vi "Dashboard Main.vi"() -> ()   [LabVIEW 2014]
uses:
  <vilib>/event_ctls.llb/eventvkey.ctl
  <vilib>/Rock Robotics/WPI/Dashboard/WPI_DashboardLogging Global.vi
  <vilib>/Rock Robotics/Network Tables/SD Write Numeric Array.vi
  <vilib>/Rock Robotics/Network Tables/SD Write String.vi
  <vilib>/Rock Robotics/Network Tables/SD Read Number.vi
  <vilib>/Utility/config.llb/Write Key (String).vi
  <vilib>/Utility/config.llb/Write Key (I32).vi
  <vilib>/Utility/config.llb/NI_LVConfig.lvlib
panel:
  in  "TCP":refnum<k5>
  in  "Rec Mode":enum32{"Stop", "Record", "Playback"}(radio)
  in  "Vision":u16(ring) items=["Camera Off", "USB Camera SW", "USB Camera HW", "IP Camera"]
  out "Camera IP":string
  out "Image Message":string="Timeout in Camera Communications"
  in  "Dashboard Tab":T1(tab)
  in  "Camera Settings":T2={"Frame Rate"=30, "Compression"=30, "Size"=1} {"Frame Rate" scale=1.0..30.0; "Size" items=["640x480", "320x240", "160x120"]}
  out "MotorChart R":cluster{"Numeric":dbl, "Numeric":dbl}(graph)
  out "MotorChart L":T3(graph)
  out "MotorSliders R":cluster{"MotorSlide1":dbl, "MotorSlide2":dbl} {"MotorSlide2" scale=-1.0..1.0 scale format="%#_2e"; "MotorSlide1" scale=-1.0..1.0 scale format="%#_2e"}
  out "MotorSliders L":T4 {"MotorSlide4 2" scale=0.0..14.0 scale format="%#_2e"; "MotorSlide2" scale=-1.0..1.0 scale format="%#_2e"; "MotorSlide1" scale=-1.0..1.0 scale format="%#_2e"}
  out "Gyro":dbl(knob) scale=0.0..360.0
  out "JS1 Z":dbl(slide) scale=-1.0..1.0 scale format="%#_2e"
  out "JS1 Graph":cluster{"X":dbl, "Y":dbl}[](graph)
  out "JS1 Buttons":T5
  out "JS2 Z":dbl(slide) scale=-1.0..1.0 scale format="%#_2e"
  out "JS2 Graph":cluster{"X":dbl, "Y":dbl}[](graph)
  out "JS2 Buttons":T5
  out "Mode":T6(ring)=enum."Auto Disabled"
  in  "DB Camera Config":bool
  out "fps":dbl format="%#.1g"
  out "Mbps":dbl format="%#.1g"
  out "Mbps 2":bool
  in  "DB/String 9":string
  in  "DB/String 8":string
  in  "DB/String 7":string
  in  "DB/String 6":string
  in  "DB/String 5":string
  in  "DB/String 4":string
  in  "DB/String 3":string
  in  "DB/String 2":string
  in  "DB/String 1":string
  in  "DB/String 0":string
  in  "DB/Slider 0":dbl(slide) scale=0.0..5.0
  in  "DB/Slider 1":dbl(slide) scale=0.0..5.0
  in  "DB/Slider 2":dbl(slide) scale=0.0..5.0
  in  "DB/Slider 3":dbl(slide) scale=0.0..5.0
  out "DB/LED 3":bool
  out "DB/LED 2":bool
  out "DB/LED 1":bool
  out "DB/LED 0":bool
  in  "DB/Button 3":bool
  in  "DB/Button 2":bool
  in  "DB/Button 1":bool
  in  "DB/Button 0":bool caption="New Name"
  in  "Turning Speed":dbl
  in  "Initial turn (Degrees)":dbl
  in  "Move Speed":dbl
  in  "Arm Speed":dbl
  in  "Shifting Speed":dbl
  in  "Desired Arm height (Lift)":dbl
  in  "Desired Arm height (Lowered)":dbl
  in  "Shifting time (Initial)":dbl
  in  "Auto Mode":string(combo)
  in  "Test Slider":dbl(slide) scale=0.0..100.0 scale format="%#_3g"
  in  "On/Off":bool caption="Solenoid"
  in  "Test Name":u16(ring) items=["Select the test to run...", "Example Test", "-------------------------------", "List of tests is built in robot code.", "Replace with your own automated tests."]
  in  "Test Tree":string(tree)
  in  "Motor":cluster{"Value":dbl, "Enable":bool} {"Value" scale=-1.0..1.0 scale format="%#_3g"}
  out "Progress":T7 {"Test Progress" scale=0.0..100.0}
  in  "Rev/Fwd":cluster{"Forward":bool, "Reverse":bool}
  in  "Test Ring":u16(ring) items=["Monochrome", "Color"]
  in  "Listbox":i32(listbox)
  out "Tree":string(tree)
  out "Camera Image":T8(plugin-control)
  out "Boolean":bool
  # "Left"
  # "Front"
  # "Right"
  # "Battery"
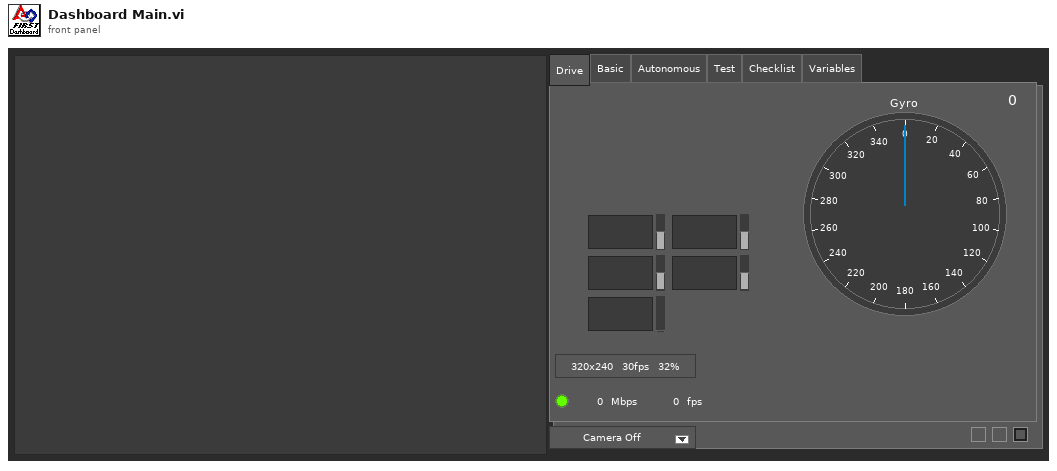
[diagram p1: front panel]
types:
  T1 = enum32{"Drive", "Basic", "Autonomous", "Test", "Checklist", "Variables"}
  T2 = cluster{"Frame Rate":i32, "Compression":i32, "Size":u16}
  T3 = cluster{"Numeric":dbl, "Numeric":dbl, "Battery V":dbl}
  T4 = cluster{"MotorSlide1":dbl, "MotorSlide2":dbl, "MotorSlide4 2":dbl}
  T5 = cluster{bool, bool, bool, bool, bool, bool, bool, bool, bool, bool, bool, bool}
  T6 = enum8{"Tele-Op Disabled", "Tele-Op Enabled", "Auto Disabled", "Auto Enabled", "Test Disabled", "Test Enabled", "Disconnected", "No Code", "E-Stop"}
  T7 = cluster{"Test Progress":u8, "Test Progress Text":string}
  T8 = typedef "IMAQ Image.ctl" = refnum<image>
  T9 = enum32{"Drive", "Basic", "Custom", "Test", "Checklist", "Variables"}
  T10 = typedef "Image Type" = u32
  T11 = cluster{"Camera Image":refnum<vi>, "Dashboard Tab":refnum<vi>, "Boolean":refnum<vi>, "Vision":refnum<vi>, "Rec Mode":refnum<vi>, "Test Slider":refnum<vi>, "On/Off ":refnum<vi>, "Test Ring":refnum<vi>, "Rev/Fwd":refnum<vi>, "Test Name":refnum<vi>, "Motor":refnum<vi>, "Progress":refnum<vi>, "CheckList":refnum<vi>, "Tree":refnum<vi>, "Test Tree":refnum<vi>}
  T12 = cluster{"Error Strings":string, "Disable Counts":cluster{u16, u16}, "Rail Faults":cluster{u16, u16, u16}, "Robot IP":string, "DB Mode":u8, "Event Info":cluster{"Name":string, "Type":u8, "Number":u16, "Replay":u8}, "Camera Addr":string}
  T13 = cluster{"Storage":cluster{"Disk Free":u64, "RAM Block":u32, "RAM free":u32}, "CPU Utilization":cluster{"CPU % ISR":sgl, "CPU % Time Crit":sgl, "CPU % Timed Str":sgl, "CPU % High":sgl, "CPU % Above":sgl, "CPU % Normal":sgl, "CPU % Low":sgl}, "CAN":cluster{"% Bus Utilization":sgl, "Bus Off Cnt":u32, "TX_FIFO Full Cnt":u32, "Receive Error Cnt":u8, "Transmit Error Cnt":u8}, "HID":cluster{"HID Outputs":u32, "Rumble Low":u16, "Rumble High":u16}[]}
  T14 = cluster{"Status bits":cluster{"Test Mode":bool, "Autonomous":bool, "Enabled":bool, "Code Start":bool, "Brownout":bool, "Reserved 2":bool, "Reserved 3":bool, "E-Stop":bool}, "Code Trace":cluster{"Disabled":bool, "TeleOp":bool, "Auto":bool, "Test":bool}, "Controller Type":enum16{"unknown", "cRIO", "roboRio"}, "Code?":enum16{"unknown", "noCode", "code"}, "Battery V":dbl}
  T15 = cluster{"Control Bits":cluster{"TestMode":bool, "Autonomous":bool, "Enabled":bool, "FMS Present":bool, bool, bool, bool, "E-Stop":bool}, "Team Station ":u8, "Countdown":sgl, "Joystick Values":cluster{"Axes":dbl[], "Buttons":bool[], "POVs":i16[]}[]}
  T16 = cluster{"Axes":dbl[], "Buttons":bool[], "POVs":i16[]}[]
  T17 = cluster{"Axes":dbl[], "Buttons":bool[], "POVs":i16[]}
  T18 = cluster{"Buttons[0]":bool, "Buttons[1]":bool, "Buttons[2]":bool, "Buttons[3]":bool, "Buttons[4]":bool, "Buttons[5]":bool, "Buttons[6]":bool, "Buttons[7]":bool, "Buttons[8]":bool, "Buttons[9]":bool, "Buttons[10]":bool, "Buttons[11]":bool}
  T19 = typedef "NI_LVConfig.lvlib/Config Data RefNum.ctl" = refnum<k1>
  T20 = cluster{"Operation":enum16{"Update", "Clear"}, "Color Box":u32}[]
  T21 = typedef "eventvkey.ctl" = enum16{"ASCII", "Enter", "Return", "Shift", "Ctrl", "Alt", "Cmd", "Opt", "Caps", "NumLock", "Clear", "Break", "Up", "Down", "Left", "Right", "Insert", "Delete", "Home", "End", "PageUp", "PageDown", "Escape", "Help", "Pause", "ScrollLock", "F1", "F2", "F3", "F4", "F5", "F6", "F7", "F8", "F9", "F10", "F11", "F12", "F13", "F14", "F15", "F16", "F17", "F18", "F19", "F20", "F21", "F22", "F23", "F24", "Play", "VolumeUp", "VolumeDown", "Mute", "Two Byte Char"}
  T22 = cluster{"Image Size":bool, "Image Type":bool, "Pixel Value":bool, "ROI Information":bool, "Zoom Factor":bool}
  T23 = enum8{"Enabled", "Disabled", "Disabled and Grayed Out"}
  T24 = cluster{"Operation":enum16{"Update", "Clear"}, "Color Box":u32}
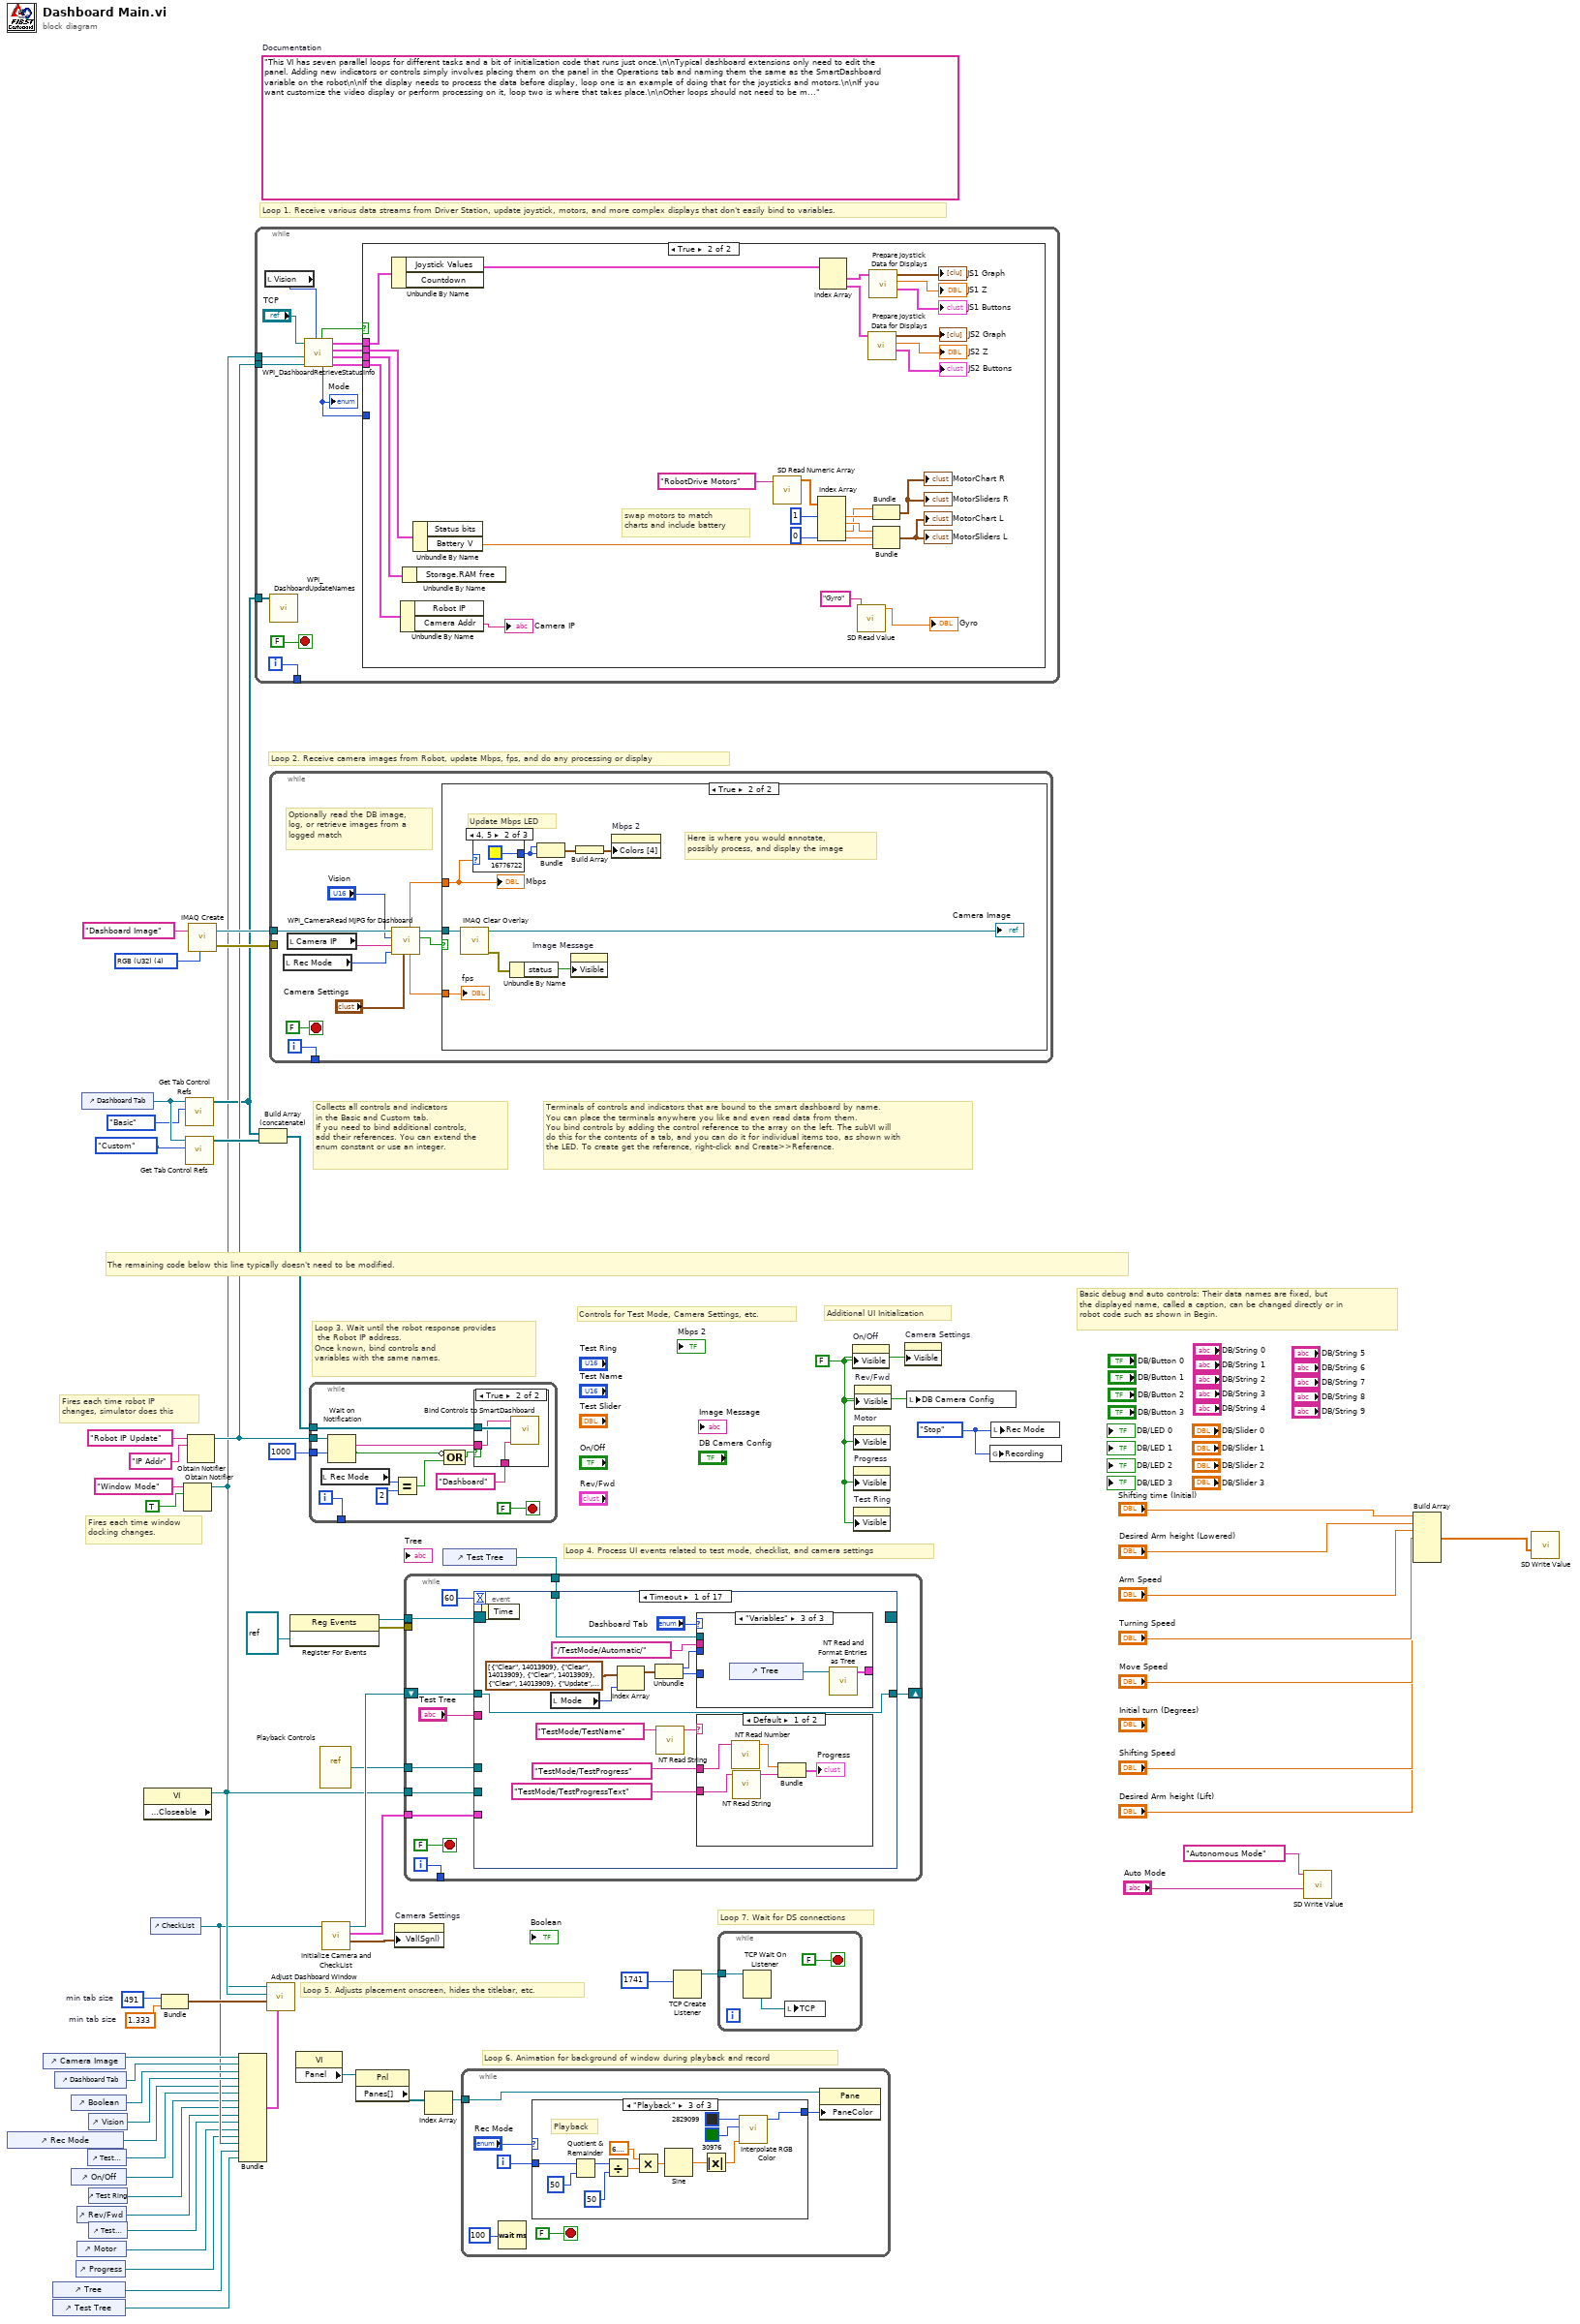
[diagram p0: block diagram]
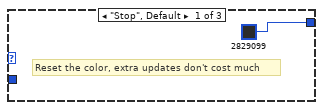
[diagram p3: hidden frame]
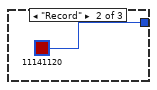
[diagram p4: hidden frame]
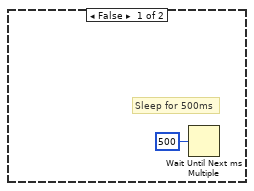
[diagram p6: hidden frame]
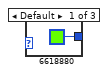
[diagram p7: hidden frame]
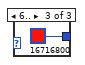
[diagram p8: hidden frame]
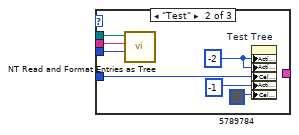
[diagram p10: hidden frame]
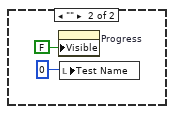
[diagram p11: hidden frame]
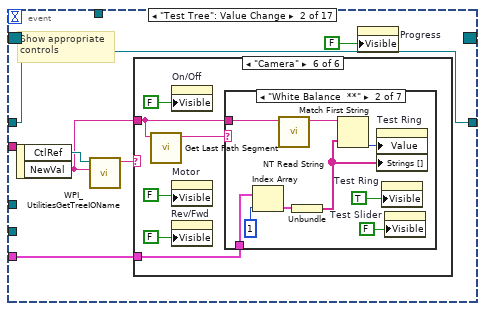
[diagram p12: hidden frame]
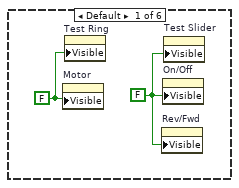
[diagram p13: hidden frame]
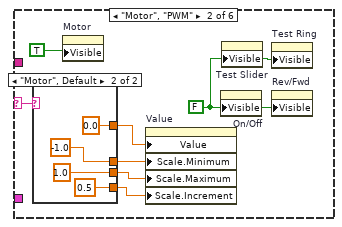
[diagram p14: hidden frame]
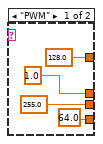
[diagram p15: hidden frame]
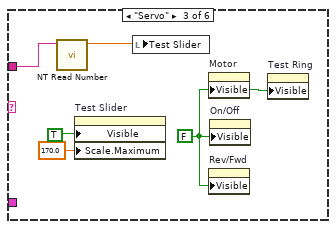
[diagram p16: hidden frame]
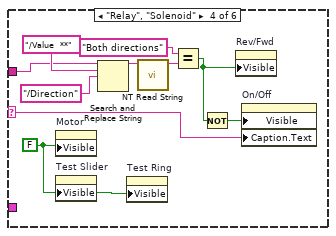
[diagram p17: hidden frame]
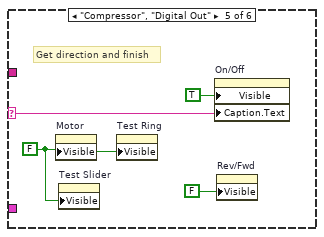
[diagram p18: hidden frame]
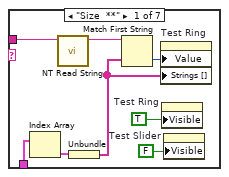
[diagram p19: hidden frame]
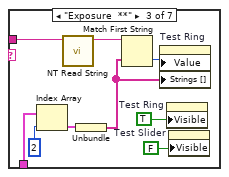
[diagram p20: hidden frame]
diagram:
  w34 = 491  # min tab size
  w33 = 1.333  # min tab size
  w42 = enum32{"Stop", "Record", "Playback"}."Stop" ("Rec Mode")
  w16 = FALSE ("Visible")
  (unwired) "This VI has seven parallel loops for different tasks and a bit of initialization code that runs just once.\n\nTypical dashboard extensions only need to edit the panel. Adding new indicators or controls simply involves placing them on the panel in the Operations tab and naming them the same as the SmartDashboard variable on the robot\n\nIf the display needs to process the data before display, loop one is an example of doing that for the joysticks and motors.\n\nIf you want customize the video display or perform processing on it, loop two is where that takes place.\n\nOther loops should not need to be modified. They are pretty standard, and document the task they perform."  # Documentation
  w62 = T10 4 items=["Grayscale (U8)", "Grayscale (I16)", "Grayscale (SGL)", "Complex (CSG)", "RGB (U32)", "HSL (U32)", "RGB (U64)"] ("Image Type")
  # "Loop 7. Wait for DS connections"
  # "Basic debug and auto controls: Their data names are fixed, but\nthe displayed name, called a caption, can be changed directly or in\nrobot code such as shown in Begin."
  # "Controls for Test Mode, Camera Settings, etc."
  # "Additional UI Initialization"
  # "Loop 6. Animation for background of window during playback and record"
  # "Fires each time robot IP\nchanges, simulator does this"
  # "Fires each time window\ndocking changes."
  # "Collects all controls and indicators\nin the Basic and Custom tab.\nIf you need to bind additional controls,\nadd their references. You can extend the\nenum constant or use an integer."
  # "The remaining code below this line typically doesn't need to be modified."
  # "Loop 4. Process UI events related to test mode, checklist, and camera settings"
  # "Terminals of controls and indicators that are bound to the smart dashboard by name.\nYou can place the terminals anywhere you like and even read data from them.\nYou bind controls by adding the control reference to the array on the left. The subVI will\ndo this for the contents of a tab, and you can do it for individual items too, as shown with\nthe LED. To create get the reference, right-click and Create>>Reference."
  # "Loop 3. Wait until the robot response provides\n the Robot IP address.\nOnce known, bind controls and\nvariables with the same names."
  # "Loop 5. Adjusts placement onscreen, hides the titlebar, etc."
  # "Loop 1. Receive various data streams from Driver Station, update joystick, motors, and more complex displays that don't easily bind to variables."
  # "Loop 2. Receive camera images from Robot, update Mbps, fps, and do any processing or display"
  n1 = control-ref of="Rec Mode"() -> (w22:refnum<vi>)
  n2 = control-ref of="Camera Image"() -> (w37:refnum<vi>)
  n3 = control-ref of="Tree"() -> (w26:refnum<vi>)
  n4 = control-ref of="Test Tree"() -> (w25:refnum<vi>)
  n5 = control-ref of="Dashboard Tab"() -> (w36:refnum<vi>)
  n6 = control-ref of="Boolean"() -> (w31:refnum<vi>)
  n7 = control-ref of="On/Off"() -> (w20:refnum<vi>)
  n8 = control-ref of="Progress"() -> (w17:refnum<vi>)
  n9 = control-ref of="Rev/Fwd"() -> (w18:refnum<vi>)
  n10 = control-ref of="Motor"() -> (w23:refnum<vi>)
  n11 = control-ref of="Dashboard Tab"() -> (w40:refnum<vi>)
  n12 = control-ref of="Test Slider"() -> (w21:refnum<vi>)
  n13 = control-ref of="Vision"() -> (w35:refnum<vi>)
  n14 = control-ref of="Test Ring"() -> (w19:refnum<vi>)
  n15 = control-ref of="Test Name"() -> (w24:refnum<vi>)
  n16 = property class="VI" props=["Front Panel.Closeable"]() -> (reference out=w41:refnum<vi>)  [unwired: 2 in, 2 out]
  n17 = control-ref of="CheckList"() -> (w27:refnum<vi>)
  n18 = Bundle("min tab size"=w34, "min tab size"=w33) -> (w32:cluster{"min tab size":i32, "min tab size":dbl})  [unwired: 1 in]
  n19 = Obtain Notifier(name (unnamed)="Window Mode", notification data type=TRUE) -> (notifier out=w13:refnum<notifier>)  [unwired: 2 in, 2 out]
  n20 = call <vilib>:"Get Tab Control Refs.vi"("Page Index"=T9."Basic" ("Dashboard Tab"), "TabControl in"=w40) -> ("ControlsOnPage"=w14:refnum<vi>[])  [unwired: 9 in]
  n21 = call <vilib>:"Get Tab Control Refs.vi"("Page Index"=T9."Custom" ("Dashboard Tab"), "TabControl in"=w40) -> ("ControlsOnPage"=w39:refnum<vi>[])  [unwired: 9 in]
  n22 = Obtain Notifier(name (unnamed)="Robot IP Update", notification data type="IP Addr" ("name (unnamed)")) -> (notifier out=w15:refnum<notifier>)  [unwired: 2 in, 2 out]
  n23 = call "IMAQ Create"("Image Name"="Dashboard Image", "Image Type"=w62) -> ("New Image"=w60:T8, "error out"=w59:errorcluster)  [unwired: 2 in, 1 out]
  n24 = Bundle("Camera Image"=w37, "Dashboard Tab"=w36, "Boolean"=w31, "Vision"=w35, "Rec Mode"=w22, "Test Slider"=w21, "On/Off"=w20, "Test Ring"=w19, "Rev/Fwd"=w18, "Test Name"=w24, "Motor"=w23, "Progress"=w17, "CheckList"=w27, "Tree"=w26, "Test Tree"=w25) -> (w28:T11)  [unwired: 1 in]
  n25 = while {
    tunnel: [w74] -> _
    tunnel: w15 -> [w68]
    tunnel: w14 -> [w67]
    tunnel: w13 -> [w63]
    i -> [w74]
    stop <- FALSE stop-if-true
    n26 = local read "Vision"() -> (w65:u16)
    n27 = call <vilib>:"WPI_DashboardUpdateNames.vi"("Controls on Tab"=w67) -> ()  [unwired: 11 in]
    n28 = call <vilib>:"WPI_DashboardRetrieveStatusInfo.vi"("Vision"=w65, "Binding Refnum"=w68, "Window Mode Notifier"=w63, "TCP Cnx"="TCP") -> ("Power and Errors"=w69:T12, "Robot Metrics"=w72:T13, "Status Info"=w73:T14, "Control Info"=w70:T15, "Robot Mode"=w66:T6, "Process?"=w71:bool)  [unwired: 2 in]
    "Mode" <- w66
    n29 = case shown="True" w71 {
      tunnel: w73 -> [_ w102]
      tunnel: w72 -> [_ w101]
      tunnel: w70 -> [_ w100]
      tunnel: w69 -> [_ w99]
      tunnel: w66 -> [_ _]
      frame False {
      }
      frame True {
        # "swap motors to match\ncharts and include battery"
        n30 = Unbundle By Name(w100) -> ("Joystick Values"=w87:T16)  [unwired: 1 out]
        n31 = Unbundle By Name(w99) -> ("Camera Addr"=→"Camera IP":string)  [unwired: 1 out]
        n32 = Unbundle By Name(w101) -> ()  [unwired: 1 out]
        n33 = Unbundle By Name(w102) -> ("Battery V"=w88:dbl)  [unwired: 1 out]
        n34 = call <vilib>:"SD Read Numeric Array.vi"("Name"="RobotDrive Motors") -> ("Numeric Array"=w90:dbl[])  [unwired: 8 in, 2 out]
        n35 = Index Array(array=w90, index #1=1, index #4=0) -> (element #1=w94:dbl, element #2=w95:dbl, element #3=w93:dbl, element #4=w98:dbl)  [unwired: 2 in]
        n36 = Index Array(array=w87) -> (element #1=w86:T17, element #2=w81:T17)  [unwired: 2 in]
        n37 = call-poly <vilib>:"SD Read Value.vi"("Name"="Gyro") -> ("Numeric"=→"Gyro":dbl)  [unwired: 8 in, 2 out]
        n38 = call "Prepare Joystick Data for Displays.vi"("Joystick Values"=w81) -> ("Buttons"=→"JS2 Buttons":T18, "Z Axis"=→"JS2 Z":dbl, "Cartesian Data"=→"JS2 Graph":cluster{"X axis":dbl, "X axis":dbl}[])  [unwired: 8 in]
        n39 = call "Prepare Joystick Data for Displays.vi"("Joystick Values"=w86) -> ("Buttons"=→"JS1 Buttons":T18, "Z Axis"=→"JS1 Z":dbl, "Cartesian Data"=→"JS1 Graph":cluster{"X axis":dbl, "X axis":dbl}[])  [unwired: 8 in]
        n40 = Bundle("Numeric"=w93, "Numeric"=w94) -> (→"MotorChart R" →"MotorSliders R":cluster{"Numeric":dbl, "Numeric":dbl})  [unwired: 1 in]
        n41 = Bundle("Numeric"=w95, "Numeric"=w98, "Battery V"=w88) -> (→"MotorChart L" →"MotorSliders L":T3)  [unwired: 1 in]
      }
    }
  }
  n42 = Build Array (concatenate)(w14, w39) -> (w38:refnum<vi>[])
  n43 = call "Adjust Dashboard Window.vi"("Sizing Refnums"=w28, "Size Constraints"=w32, "VI"=w41, "Notifier in"=w13) -> ()  [unwired: 8 in]
  n44 = while {
    tunnel: w60 -> [w111]
    tunnel: w59 -> [_]
    tunnel: [w112] -> _
    i -> [w112]
    stop <- FALSE stop-if-true
    # "Optionally read the DB image,\nlog, or retrieve images from a\nlogged match"
    n45 = local read "Rec Mode"() -> (w105:enum32{"Stop", "Record", "Playback"})
    n46 = local read "Camera IP"() -> (w103:string)
    n47 = call <vilib>:"WPI_CameraRead MJPG for Dashboard.vi"("Camera Settings"="Camera Settings", "Rec Mode"=w105, "Camera IP"=w103, "Camera Mode"="Vision", "Refnum in"=w111) -> ("Active"=w109:bool, "Refnum out"=w110:T8, "FPS"=w108:dbl, "Bandwidth (Mbps)"=w107:dbl)  [unwired: 3 in]
    n48 = case shown="True" w109 {
      tunnel: w110 -> [_ w118]
      tunnel: w107 -> [_ w117]
      tunnel: w108 -> [_ w115]
      frame False {
        # "Sleep for 500ms"
        n49 = Wait Until Next ms Multiple(millisecond multiple=u32 500) -> ()  [unwired: 1 out]
      }
      frame True {
        # "Here is where you would annotate,\npossibly process, and display the image"
        # "Update Mbps LED"
        n50 = call "IMAQ Clear Overlay"("Image"=w118) -> ("error out"=w122:errorcluster, "Image Out"=→"Camera Image":T8)  [unwired: 2 in, 7 out]
        n51 = case shown="4, 5" w117 {
          tunnel: [u32 6618880 ("Color Box") u32 16776722 ("Color Box") u32 16716800 ("Color Box")] -> w119
          frame Default {
          }
          frame 4, 5 {
          }
          frame 6.. {
          }
        }
        n52 = Unbundle By Name(w122) -> ("status"=w123:bool)
        n53 = Bundle("Color Box"=w119, "Color Box"=w119) -> (w121:cluster{"Color Box":u32, "Color Box":u32})  [unwired: 1 out]
        n54 = property on="Image Message" class="Str"("Visible"=w123) -> ()  [unwired: 2 in, 2 out]
        n55 = Build Array(w121) -> (w120:cluster{"Color Box":u32, "Color Box":u32}[])
        n56 = property on="Mbps 2" class="Bool (strict)"("Colors [4]"=w120) -> ()  [unwired: 2 in, 2 out]
        "Mbps" <- w117
        "fps" <- w115
      }
    }
  }
  n57 = register-events(refnum<vi> refnum) -> (reference out=w46:refnum<event-registration>, error out=w45:errorcluster)  [unwired: 2 in]
  n58 = property class="VI"() -> ("Panel"=w49:refnum<vi>)  [unwired: 2 in, 2 out]
  n59 = while {
    tunnel: w38 -> [w138]
    tunnel: w15 -> [w136]
    tunnel: [w134] -> _
    tunnel: u32 1000 ("milliseconds to wait") -> [w133]
    i -> [w134]
    stop <- FALSE stop-if-true
    n60 = local read "Rec Mode"() -> (w129:enum32{"Stop", "Record", "Playback"})
    n61 = Wait on Notification(notifier=w136, timeout in ms (-1)=w133) -> (notification=w135:string, timed out?=w131:bool)  [unwired: 2 in, 2 out]
    n62 = Equal?(x=w129, y=u16 2 ("Rec Mode")) -> (x = y?=w130:bool)
    n63 = Compound Arithmetic op=OR(invert w131, w130) -> (w132:bool)
    n64 = case shown="True" w132 {
      tunnel: w138 -> [_ w141]
      tunnel: w135 -> [_ w140]
      tunnel: "Dashboard" -> [_ w139]
      frame False {
      }
      frame True {
        n65 = call <vilib>:"Bind Controls to SmartDashboard.vi"("Client Name"=w139, "Bound Control Refs"=w141, "Server IP Address"=w140) -> ()  [unwired: 9 in]
      }
    }
  }
  n66 = vi-ref "Playback Controls.vi"() -> (w47:refnum<vi>)
  n67 = call "Initialize Camera and CheckList.vi"("ListBox in"=w27) -> ("Cluster"=w53:cluster{"value":i32, "value":i32, "index":i32}, "Array"=w54:cluster{string[]}[], "File Refnum"=w52:T19)  [unwired: 8 in]
  n68 = property class="Pnl"(reference=w49) -> ("Panes[]"=w50:refnum<vi>[])  [unwired: 1 in, 2 out]
  n69 = property on="Camera Settings" class="Clust (strict)"("Val(Sgnl)"=w53) -> ()  [unwired: 2 in, 2 out]
  n70 = Index Array(array=w50) -> (element=w48:refnum<vi>)  [unwired: 1 in]
  n71 = control-ref of="Test Tree"() -> (w51:refnum<vi>)
  n72 = while {
    tunnel: w54 -> [w149]
    shift-right: [w148] -> _
    shift-left: w52 -> [w147]
    tunnel: [w146] -> _
    tunnel: w51 -> [w145]
    tunnel: w47 -> [w144]
    tunnel: w46 -> [w143]
    tunnel: w45 -> [_]
    tunnel: w41 -> [w142]
    i -> [w146]
    stop <- FALSE stop-if-true
    n73 = event shown="[0] Timeout" {
      selector: w143 -> [_ _ _ _ _ _ _ _ _ _ _ _ _ _ _ _ _]
      dyn-events: [_ _ _ _ _ _ _ _ _ _ _ _ _ w387 _ _ _] -> _
      timeout: u32 60 ("milliseconds to wait") -> [_ _ _ _ _ _ _ _ _ _ _ _ _ _ _ _ _]
      tunnel: w145 -> [w161 _ _ _ _ _ _ _ _ _ _ _ _ _ _ _ _]
      tunnel: "Test Tree" -> [_ _ _ _ _ _ _ _ w356 w364 w366 w370 w378 _ _ _ _]
      tunnel: w149 -> [_ w183 _ _ _ _ w320 w350 _ _ _ _ _ _ _ _ _]
      tunnel: [w157 w182 w281 w286 w294 w306 w319 w343 w355 w362 w365 w369 w377 w389 w403 w404 w414] -> w148
      tunnel: w147 -> [w157 w182 w281 w286 w294 w306 w318 w343 w355 w362 w365 w369 w377 w389 w403 w404 w414]
      tunnel: w144 -> [_ _ _ _ _ _ _ _ _ _ _ _ _ w390 _ w407 _]
      tunnel: w142 -> [_ _ _ _ _ _ _ _ _ _ _ _ _ w385 _ _ _]
      event Timeout {
        n74 = event-data() -> ()  [unwired: 1 in, 1 out]
        n75 = local read "Mode"() -> (w160:T6)
        n76 = Index Array(array=T20 [{"Operation"=enum."Clear", "Color Box"=14013909}, {"Operation"=enum."Clear", "Color Box"=14013909}, {"Operation"=enum."Clear", "Color Box"=14013909}, {"Operation"=enum."Clear", "Color Box"=14013909}, {"Operation"=enum."Update", "Color Box"=14013909}, {"Operation"=enum."Update", "Color Box"=16777215}, {"Operation"=enum."Clear", "Color Box"=14013909}, {"Operation"=enum."Clear", "Color Box"=14013909}, {"Operation"=enum."Clear", "Color Box"=14013909}], index=w160) -> (element=w155:T24)
        n77 = Unbundle(w155) -> ("Operation"=w154:enum16{"Update", "Clear"}, "Color Box"=w153:u32)
        n78 = call <vilib>:"NT Read String.vi"("Name"="TestMode/TestName") -> ("String"=w164:string)  [unwired: 9 in, 1 out]
        n79 = case shown="\"Variables\"" "Dashboard Tab" {
          tunnel: w161 -> [_ w172 _]
          tunnel: "/TestMode/Automatic/" ("Name Pattern") -> [_ w171 _]
          tunnel: w154 -> [_ w170 _]
          tunnel: [_ _ w174] -> _
          tunnel: w153 -> [_ w166 _]
          frame "Autonomous", Default {
          }
          frame "Test" {
            w169 = -2 ("Active Item:Row Number")
            n80 = call <vilib>:"NT Read and Format Entries as Tree.vi"("Operation"=w170, "Name Pattern"=w171, "Tree Refnum"=w172) -> ()  [unwired: 7 in, 2 out]
            n81 = property on="Test Tree" class="Tree (strict)"("Active Item Row Number"=w169, "ActiveColNum"=w169, "CellBG"=w166, "Active Item Row Number"=-1 ("Active Item:Row Number"), "CellBG"=u32 5789784 ("Color Box")) -> ()  [unwired: 2 in, 2 out]
          }
          frame "Variables" {
            n82 = control-ref of="Tree"() -> (w173:refnum<vi>)
            n83 = call <vilib>:"NT Read and Format Entries as Tree.vi"("Tree Refnum"=w173) -> ("Formatted Strings"=w174:cluster{"Name":string, "Value":string}[])  [unwired: 9 in, 1 out]
          }
        }
        n84 = case shown="Default" w164 {
          tunnel: "TestMode/TestProgress" ("Name") -> [w176 _]
          tunnel: "TestMode/TestProgressText" ("Name") -> [w175 _]
          frame Default {
            n85 = call <vilib>:"NT Read Number.vi"("Name"=w176) -> ("Numeric"=w177:dbl)  [unwired: 9 in, 1 out]
            n86 = call <vilib>:"NT Read String.vi"("Name"=w175) -> ("String"=w178:string)  [unwired: 9 in, 1 out]
            n87 = Bundle("Numeric"=w177, "String"=w178) -> (→"Progress":cluster{"Numeric":dbl, "String":string})  [unwired: 1 in]
          }
          frame "" {
            n88 = property on="Progress" class="Clust (strict)"("Visible"=FALSE) -> ()  [unwired: 2 in, 2 out]
            n89 = local write "Test Name"(u16 0) -> ()
          }
        }
      }
      event "Test Tree": Value Change {
        # "Show appropriate\ncontrols"
        n90 = event-data() -> ("CtlRef"=w186:refnum<vi>, "NewVal"=w184:string)  [unwired: 1 in]
        n91 = call <vilib>:"WPI_UtilitiesGetTreeIOName.vi"("NewVal"=w184, "TreeControl in"=w186) -> ("I/O Name"=w187:string)  [unwired: 9 in]
        n92 = case shown="\"Camera\"" w187 {
          selector: w187 -> [_ w194 _ w212 w221 _]
          tunnel: w184 -> [_ _ w209 w211 _ w228]
          tunnel: w183 -> [_ _ _ _ _ w227]
          frame Default {
            w189 = FALSE ("Visible")
            w188 = FALSE ("Visible")
            n93 = property on="Motor" class="Clust (strict)"("Visible"=w188) -> ()  [unwired: 2 in, 2 out]
            n94 = property on="Test Ring" class="Ring (strict)"("Visible"=w188) -> ()  [unwired: 2 in, 2 out]
            n95 = property on="Rev/Fwd" class="Clust (strict)"("Visible"=w189) -> ()  [unwired: 2 in, 2 out]
            n96 = property on="On/Off" class="Bool (strict)"("Visible"=w189) -> ()  [unwired: 2 in, 2 out]
            n97 = property on="Test Slider" class="Slide (strict)"("Visible"=w189) -> ()  [unwired: 2 in, 2 out]
          }
          frame "Motor", "PWM" {
            w195 = FALSE ("Visible")
            n98 = case shown="\"Motor\", Default" w194 {
              tunnel: [1.0 ("Value") -1.0 ("Value")] -> w193
              tunnel: [255.0 ("Value") 1.0 ("Value")] -> w192
              tunnel: [128.0 ("Value") 0.0 ("Value")] -> w191
              tunnel: [64.0 ("Value") 0.5 ("Value")] -> w190
              frame "PWM" {
              }
              frame "Motor", Default {
              }
            }
            n99 = property on="Motor" class="Clust (strict)"("Visible"=TRUE) -> ()  [unwired: 2 in, 2 out]
            n100 = property on="Value" class="Slide (strict)"("Value"=w191, "Scale.Minimum"=w193, "Scale.Maximum"=w192, "Scale.Increment"=w190) -> ()  [unwired: 2 in, 2 out]
            n101 = property on="On/Off" class="Bool (strict)"("Visible"=w195) -> ()  [unwired: 2 in, 2 out]
            n102 = property on="Test Slider" class="Slide (strict)"("Visible"=w195) -> ()  [unwired: 2 in, 2 out]
            n103 = property on="Test Ring" class="Ring (strict)"("Visible"=w195) -> ()  [unwired: 2 in, 2 out]
            n104 = property on="Rev/Fwd" class="Clust (strict)"("Visible"=w195) -> ()  [unwired: 2 in, 2 out]
          }
          frame "Servo" {
            w207 = FALSE ("Visible")
            n105 = call <vilib>:"NT Read Number.vi"("Name"=w209) -> ("Numeric"=w208:dbl)  [unwired: 9 in, 1 out]
            n106 = property on="Test Slider" class="Slide (strict)"("Visible"=TRUE, "Scale.Maximum"=170.0 ("Scale.Range:Maximum")) -> ()  [unwired: 2 in, 2 out]
            n107 = local write "Test Slider"(w208) -> ()
            n108 = property on="Motor" class="Clust (strict)"("Visible"=w207) -> ()  [unwired: 2 in, 2 out]
            n109 = property on="Rev/Fwd" class="Clust (strict)"("Visible"=w207) -> ()  [unwired: 2 in, 2 out]
            n110 = property on="On/Off" class="Bool (strict)"("Visible"=w207) -> ()  [unwired: 2 in, 2 out]
            n111 = property on="Test Ring" class="Ring (strict)"("Visible"=w207) -> ()  [unwired: 2 in, 2 out]
          }
          frame "Relay", "Solenoid" {
            w210 = FALSE ("Visible")
            n112 = property on="Motor" class="Clust (strict)"("Visible"=w210) -> ()  [unwired: 2 in, 2 out]
            n113 = property on="Test Slider" class="Slide (strict)"("Visible"=w210) -> ()  [unwired: 2 in, 2 out]
            n114 = Search and Replace String(input string=w211, search string="/Value  **", replace string="/Direction") -> (result string=w217:string)  [unwired: 5 in, 3 out]
            n115 = property on="Test Ring" class="Ring (strict)"("Visible"=w210) -> ()  [unwired: 2 in, 2 out]
            n116 = call <vilib>:"NT Read String.vi"("Name"=w217) -> ("String"=w215:string)  [unwired: 9 in, 1 out]
            n117 = Equal?(x="Both directions", y=w215) -> (x = y?=w213:bool)
            n118 = Not(x=w213) -> (.not. x?=w214:bool)
            n119 = property on="Rev/Fwd" class="Clust (strict)"("Visible"=w213) -> ()  [unwired: 2 in, 2 out]
            n120 = property on="On/Off" class="Bool (strict)"("Visible"=w214, "Caption.Text"=w212) -> ()  [unwired: 2 in, 2 out]
          }
          frame "Compressor", "Digital Out" {
            w220 = FALSE ("Visible")
            # "Get direction and finish"
            n121 = property on="Motor" class="Clust (strict)"("Visible"=w220) -> ()  [unwired: 2 in, 2 out]
            n122 = property on="Test Slider" class="Slide (strict)"("Visible"=w220) -> ()  [unwired: 2 in, 2 out]
            n123 = property on="Test Ring" class="Ring (strict)"("Visible"=w220) -> ()  [unwired: 2 in, 2 out]
            n124 = property on="On/Off" class="Bool (strict)"("Visible"=TRUE, "Caption.Text"=w221) -> ()  [unwired: 2 in, 2 out]
            n125 = property on="Rev/Fwd" class="Clust (strict)"("Visible"=FALSE) -> ()  [unwired: 2 in, 2 out]
          }
          frame "Camera" {
            n126 = call <vilib>:"Get Last Path Segment.vi"("String in"=w228) -> ("String out"=w229:string)  [unwired: 10 in]
            n127 = property on="On/Off" class="Bool (strict)"("Visible"=FALSE) -> ()  [unwired: 2 in, 2 out]
            n128 = property on="Motor" class="Clust (strict)"("Visible"=FALSE) -> ()  [unwired: 2 in, 2 out]
            n129 = property on="Rev/Fwd" class="Clust (strict)"("Visible"=FALSE) -> ()  [unwired: 2 in, 2 out]
            n130 = case shown="\"White Balance  **\"" w229 {
              tunnel: w228 -> [w235 w244 w253 w262 w271 _ w277]
              tunnel: w227 -> [w233 w241 w250 w259 w268 _ _]
              frame "Size  **" {
                n131 = Index Array(array=w233) -> (element=w232:cluster{string[]})  [unwired: 1 in]
                n132 = call <vilib>:"NT Read String.vi"("Name"=w235) -> ("String"=w234:string)  [unwired: 9 in, 1 out]
                n133 = Unbundle(w232) -> (w230:string[])
                n134 = Match First String(2:w230, 3:w234) -> (0:w231:i32)  [unwired: 1 out]
                n135 = property on="Test Ring" class="Ring (strict)"("Value"=w231, "Strings []"=w230) -> ()  [unwired: 2 in, 2 out]
                n136 = property on="Test Ring" class="Ring (strict)"("Visible"=TRUE) -> ()  [unwired: 2 in, 2 out]
                n137 = property on="Test Slider" class="Slide (strict)"("Visible"=FALSE) -> ()  [unwired: 2 in, 2 out]
              }
              frame "White Balance  **" {
                n138 = Index Array(array=w241, index=1) -> (element=w242:cluster{string[]})
                n139 = call <vilib>:"NT Read String.vi"("Name"=w244) -> ("String"=w243:string)  [unwired: 9 in, 1 out]
                n140 = Unbundle(w242) -> (w239:string[])
                n141 = Match First String(2:w239, 3:w243) -> (0:w238:i32)  [unwired: 1 out]
                n142 = property on="Test Ring" class="Ring (strict)"("Value"=w238, "Strings []"=w239) -> ()  [unwired: 2 in, 2 out]
                n143 = property on="Test Ring" class="Ring (strict)"("Visible"=TRUE) -> ()  [unwired: 2 in, 2 out]
                n144 = property on="Test Slider" class="Slide (strict)"("Visible"=FALSE) -> ()  [unwired: 2 in, 2 out]
              }
              frame "Exposure  **" {
                n145 = Index Array(array=w250, index=2) -> (element=w251:cluster{string[]})
                n146 = call <vilib>:"NT Read String.vi"("Name"=w253) -> ("String"=w252:string)  [unwired: 9 in, 1 out]
                n147 = Unbundle(w251) -> (w247:string[])
                n148 = Match First String(2:w247, 3:w252) -> (0:w248:i32)  [unwired: 1 out]
                n149 = property on="Test Ring" class="Ring (strict)"("Value"=w248, "Strings []"=w247) -> ()  [unwired: 2 in, 2 out]
                n150 = property on="Test Ring" class="Ring (strict)"("Visible"=TRUE) -> ()  [unwired: 2 in, 2 out]
                n151 = property on="Test Slider" class="Slide (strict)"("Visible"=FALSE) -> ()  [unwired: 2 in, 2 out]
              }
              frame "Exposure Priority  **" {
                n152 = Index Array(array=w259, index=3) -> (element=w260:cluster{string[]})
                n153 = call <vilib>:"NT Read String.vi"("Name"=w262) -> ("String"=w261:string)  [unwired: 9 in, 1 out]
                n154 = Unbundle(w260) -> (w256:string[])
                n155 = Match First String(2:w256, 3:w261) -> (0:w257:i32)  [unwired: 1 out]
                n156 = property on="Test Ring" class="Ring (strict)"("Value"=w257, "Strings []"=w256) -> ()  [unwired: 2 in, 2 out]
                n157 = property on="Test Ring" class="Ring (strict)"("Visible"=TRUE) -> ()  [unwired: 2 in, 2 out]
                n158 = property on="Test Slider" class="Slide (strict)"("Visible"=FALSE) -> ()  [unwired: 2 in, 2 out]
              }
              frame "Color Enable  **" {
                n159 = Index Array(array=w268, index=4) -> (element=w269:cluster{string[]})
                n160 = call <vilib>:"NT Read String.vi"("Name"=w271) -> ("String"=w270:string)  [unwired: 9 in, 1 out]
                n161 = Unbundle(w269) -> (w265:string[])
                n162 = Match First String(2:w265, 3:w270) -> (0:w266:i32)  [unwired: 1 out]
                n163 = property on="Test Ring" class="Ring (strict)"("Value"=w266, "Strings []"=w265) -> ()  [unwired: 2 in, 2 out]
                n164 = property on="Test Ring" class="Ring (strict)"("Visible"=TRUE) -> ()  [unwired: 2 in, 2 out]
                n165 = property on="Test Slider" class="Slide (strict)"("Visible"=FALSE) -> ()  [unwired: 2 in, 2 out]
              }
              frame Default {
                n166 = property on="Test Ring" class="Ring (strict)"("Visible"=FALSE) -> ()  [unwired: 2 in, 2 out]
                n167 = property on="Test Slider" class="Slide (strict)"("Visible"=FALSE) -> ()  [unwired: 2 in, 2 out]
              }
              frame "Brightness  **", "Color Level  **", "Compression  **", "FPS  **", "Sharpness  **" {
                n168 = call <vilib>:"NT Read Number.vi"("Name"=w277) -> ("Numeric"=w276:dbl)  [unwired: 9 in, 1 out]
                n169 = local write "Test Slider"(w276) -> ()
                n170 = property on="Test Slider" class="Slide (strict)"("Visible"=TRUE, "Scale.Maximum"=100.0 ("Scale.Range:Maximum")) -> ()  [unwired: 2 in, 2 out]
                n171 = property on="Test Ring" class="Ring (strict)"("Visible"=FALSE) -> ()  [unwired: 2 in, 2 out]
              }
            }
          }
        }
        n172 = property on="Progress" class="Clust (strict)"("Visible"=FALSE) -> ()  [unwired: 2 in, 2 out]
      }
      event "Test Name": Mouse Enter {
        # "Populate the ring with the list of tests"
        n173 = event-data() -> ()  [unwired: 1 in, 1 out]
        n174 = call <vilib>:"NT Read String Array.vi"("Name"="TestMode/TestList") -> ("String Array"=w285:string[])  [unwired: 9 in, 1 out]
        n175 = Build Array (concatenate)("Select the test to run...", w285) -> (w284:string[])
        n176 = property on="Test Name" class="Ring (strict)"("Strings []"=w284) -> ()  [unwired: 2 in, 2 out]
      }
      event "Test Name": Value Change {
        w287 = FALSE ("Visible")
        # "Tell the robot the test name to run"
        n177 = event-data() -> ("NewVal"=w291:u16)  [unwired: 1 in]
        n178 = property on="Test Name" class="Ring (strict)"() -> ("Strings []"=w292:string[])  [unwired: 2 in, 2 out]
        n179 = local write "Progress"(T7 {"Test Progress"=0, "Test Progress Text"=""} ("Progress")) -> ()
        n180 = Index Array(array=w292, index=w291) -> (element=w290:string)
        n181 = call <vilib>:"NT Write String.vi"("String"=w290, "Name"="TestMode/TestName") -> ()  [unwired: 9 in, 1 out]
        n182 = property on="Progress" class="Clust (strict)"("Visible"=TRUE) -> ()  [unwired: 2 in, 2 out]
        n183 = property on="Motor" class="Clust (strict)"("Visible"=w287) -> ()  [unwired: 2 in, 2 out]
        n184 = property on="Test Slider" class="Slide (strict)"("Visible"=w287) -> ()  [unwired: 2 in, 2 out]
        n185 = property on="On/Off" class="Bool (strict)"("Visible"=w287) -> ()  [unwired: 2 in, 2 out]
        n186 = property on="Rev/Fwd" class="Clust (strict)"("Visible"=w287) -> ()  [unwired: 2 in, 2 out]
        n187 = property on="Test Ring" class="Ring (strict)"("Visible"=w287) -> ()  [unwired: 2 in, 2 out]
      }
      event "Listbox": Double Click {
        # "Shift clears all"
        # "Update symbols on the listbox"
        n188 = event-data() -> ("PlatMods.Shift"=w295:bool, "Row"=w297:i32)  [unwired: 1 in]
        n189 = case shown="True" w295 {
          tunnel: w297 -> [w301 _]
          tunnel: 1 -> [w300 _]
          frame False {
            n190 = property on="Listbox" class="LstBox (strict)"() -> ("Item Symbols"=w299:i32[])  [unwired: 2 in, 2 out]
            n191 = Replace Array Subset(array=w299, new element=w300, index=w301) -> (w298:i32[])
            n192 = property on="Listbox" class="LstBox (strict)"("Item Symbols"=w298) -> ()  [unwired: 2 in, 2 out]
          }
          frame True {
            w302 = 0 ("Top Row")
            n193 = property on="Listbox" class="LstBox (strict)"() -> ("Number of Rows"=w304:u32)  [unwired: 2 in, 2 out]
            n194 = Initialize Array(0, w304) -> (w303:i32[])
            n195 = property on="Listbox" class="LstBox (strict)"("Top Row"=w302, "Value"=w302, "Item Symbols"=w303) -> ()  [unwired: 2 in, 2 out]
          }
        }
      }
      event "Listbox": Key Down {
        # "Update symbols on the listbox\nLeft and right keys check and uncheck"
        n196 = event-data() -> ("VKey"=w308:T21)  [unwired: 1 in]
        n197 = case shown="\"Left\", \"Right\"" w308 {
          selector: w308 -> [w313 _]
          tunnel: eventvkey."Left" ("VKey") -> [w311 _]
          frame "Left", "Right" {
            n198 = Equal?(x=w311, y=w313) -> (x = y?=w312:bool)
            n199 = Select(t=0, s=w312, f=1) -> (s? t:f=w314:i32)
            n200 = property on="Listbox" class="LstBox (strict)"() -> ("Item Symbols"=w317:i32[])  [unwired: 2 in, 2 out]
            n201 = Replace Array Subset(array=w317, new element=w314, index="Listbox") -> (w316:i32[])
            n202 = property on="Listbox" class="LstBox (strict)"("Item Symbols"=w316) -> ()  [unwired: 2 in, 2 out]
          }
          frame Default {
          }
        }
      }
      event "DB Camera Config": Value Change {
        # "Show or hide the cluster of controls, store in ini file"
        n203 = event-data() -> ("NewVal"=w321:bool)  [unwired: 1 in]
        n204 = case shown="False" w321 {
          tunnel: w320 -> [w330 _]
          tunnel: [w323 w341] -> w319
          tunnel: w318 -> [w322 w341]
          frame False {
            w337 = "Camera"
            w340 = FALSE ("Visible")
            n205 = local read "Camera Settings"() -> (w329:T2)
            n206 = Index Array(array=w330) -> (element=w333:cluster{string[]})  [unwired: 1 in]
            n207 = Unbundle(w329) -> ("Frame Rate"=w328:i32, "Compression"=w327:i32, "Size"=w331:u16)
            n208 = Unbundle(w333) -> (w332:string[])
            n209 = Index Array(array=w332, index=w331) -> (element=w326:string)
            n210 = call-poly <vilib>:"Write Key.vi"("section"=w337, "value"=w326, "key"="Size", "refnum"=w322) -> ("refnum out"=w339:T19)  [unwired: 2 in, 5 out]
            n211 = call-poly <vilib>:"Write Key.vi"("section"=w337, "value"=w328, "key"="FrameRate", "refnum"=w339) -> ("refnum out"=w338:T19)  [unwired: 1 in, 6 out]
            n212 = property on="Camera Settings" class="Clust (strict)"("Visible"=w340) -> ()  [unwired: 2 in, 2 out]
            n213 = local write "DB Camera Config"(w340) -> ()
            n214 = call-poly <vilib>:"Write Key.vi"("section"=w337, "value"=w327, "key"="Compression", "refnum"=w338) -> ("refnum out"=w324:T19)  [unwired: 1 in, 6 out]
            n215 = call <vilib>:"Close Config Data.vi"("refnum"=w324) -> ("file path"=w325:path)  [unwired: 2 in, 8 out]
            n216 = call <vilib>:"Open Config Data.vi"("configuration file path"=w325) -> ("refnum"=w323:T19)  [unwired: 8 in, 2 out]
          }
          frame True {
            n217 = property on="Camera Settings" class="Clust (strict)"("Visible"=TRUE) -> ()  [unwired: 2 in, 2 out]
          }
        }
      }
      event "Camera Settings": Value Change {
        # "Update summary string when any elements of DB camera change"
        n218 = event-data() -> ("NewVal"=w354:T2)  [unwired: 1 in]
        n219 = Index Array(array=w350) -> (element=w349:cluster{string[]})  [unwired: 1 in]
        n220 = Unbundle(w354) -> ("Frame Rate"=w345:i32, "Compression"=w344:i32, "Size"=w347:u16)
        n221 = Unbundle(w349) -> (w348:string[])
        n222 = Index Array(array=w348, index=w347) -> (element=w346:string)
        n223 = Format Into String(format string="%s   %dfps   %d%%", w346, w345, w344) -> (resulting string=w351:string)  [unwired: 2 in, 1 out]
        n224 = Build Array(w351) -> (w352:string[])
        n225 = property on="DB Camera Config" class="Bool (strict)"("Strings [4]"=w352) -> ()  [unwired: 2 in, 2 out]
      }
      event "Motor.Enable": Value Change {
        # "When the test mode otor enable helper is set, update that\ntree row item's value"
        n226 = event-data() -> ("NewVal"=w360:bool)  [unwired: 1 in]
        n227 = Unbundle("Motor") -> ("Value"=w359:dbl)  [unwired: 1 out]
        n228 = Select(t=w359, s=w360, f=0.0) -> (s? t:f=w357:dbl)
        n229 = call <vilib>:"NT Write Number.vi"("Numeric"=w357, "Name"=w356) -> ()  [unwired: 9 in, 1 out]
      }
      event "Test Slider": Value Change {
        # "When the test mode slider helper is set, update that\ntree row item's value"
        n230 = event-data() -> ("NewVal"=w363:dbl)  [unwired: 1 in]
        n231 = call <vilib>:"NT Write Number.vi"("Numeric"=w363, "Name"=w364) -> ()  [unwired: 9 in, 1 out]
      }
      event "On/Off": Value Change {
        # "When the test mode on/off helper value is set, update that\ntree row item's value"
        n232 = event-data() -> ("NewVal"=w368:bool)  [unwired: 1 in]
        n233 = Boolean To (0,1)(Boolean=w368) -> (0, 1=w367:i16)
        n234 = call <vilib>:"NT Write Number.vi"("Numeric"=w367, "Name"=w366) -> ()  [unwired: 9 in, 1 out]
      }
      event "Rev/Fwd": Value Change {
        # "When the test mode helper value for relays is set, update that\ntree row item's value"
        n235 = event-data() -> ("NewVal.Forward"=w376:bool, "NewVal.Reverse"=w375:bool)  [unwired: 1 in]
        n236 = Boolean To (0,1)(Boolean=w376) -> (0, 1=w372:i16)
        n237 = Boolean To (0,1)(Boolean=w375) -> (0, 1=w374:i16)
        n238 = Negate(x=w374) -> (-x=w373:i16)
        n239 = Add(x=w372, y=w373) -> (x+y=w371:i16)
        n240 = call <vilib>:"NT Write Number.vi"("Numeric"=w371, "Name"=w370) -> ()  [unwired: 9 in, 1 out]
      }
      event "Test Ring": Value Change {
        # "When a test mode helper value is selected from the ring,\nset the tree item's variable to the string value"
        n241 = event-data() -> ("NewVal"=w380:u16)  [unwired: 1 in]
        n242 = property on="Test Ring" class="Ring (strict)"() -> ("Strings []"=w381:string[])  [unwired: 2 in, 2 out]
        n243 = Index Array(array=w381, index=w380) -> (element=w379:string)
        n244 = call <vilib>:"NT Write String.vi"("String"=w379, "Name"=w378) -> ()  [unwired: 9 in, 1 out]
      }
      event "Rec Mode": Value Change {
        # "Update globals for recording mode and path to read log from.\nClear when logging and let NetworkTables set path for vision to\nuse."
        n245 = event-data() -> ("NewVal"=w391:enum32{"Stop", "Record", "Playback"})  [unwired: 1 in]
        n246 = global write "WPI_DashboardLogging Global.vi" "Logging Filename"(path "") -> ()
        n247 = case shown="\"Playback\"" w391 {
          tunnel: w390 -> [_ w393 w401]
          tunnel: [_ _ w400] -> w387
          tunnel: [_ _ w399] -> _
          tunnel: w385 -> [_ _ w397]
          tunnel: cluster{i32, i32} {-250, 170} -> [_ _ w396]
          tunnel: [_ _ T22 {"Image Size"=TRUE, "Image Type"=TRUE, "Pixel Value"=TRUE, "ROI Information"=TRUE, "Zoom Factor"=FALSE} ("Image Information Shown:All Elements")] -> w383
          tunnel: [_ _ TRUE ("Zoom Factor")] -> w382
          frame Default {
          }
          frame "Stop", "Record" {
            # "Place Window too"
            n248 = invoke class="VI" method="FP.Close"(reference=w393) -> (reference out=w392:refnum<vi>)  [unwired: 2 in, 2 out]
            n249 = invoke class="VI" method="Abort VI"(reference=w392) -> ()  [unwired: 2 in, 3 out]
          }
          frame "Playback" {
            n250 = call "Open Playback Panel.vi"("Offset"=w396, "DB VI Ref"=w397, "Playback in"=w401) -> ("Playback out"=w398:refnum<vi>)  [unwired: 8 in]
            n251 = register-events(w398) -> (reference out=w400:refnum<event-registration>, error out=w399:errorcluster)  [unwired: 2 in]
          }
        }
        n252 = global write "WPI_DashboardLogging Global.vi" "Recording"(w391) -> ()
        n253 = property on="Camera Image" class="ImageControl"("Image Information Shown"=w383, "Image Information Visible"=w382) -> ()  [unwired: 2 in, 2 out]
        n254 = call <vilib>:"WPI_DashboardNT Log FieldName Cache.vi"("Operation"=enum16{"Lookup/Add", "Index", "Clear"}."Clear") -> ()  [unwired: 8 in, 3 out]
      }
      event Panel Close {
        w402 = enum32{"Stop", "Record", "Playback"}."Stop" ("Rec Mode")
        # "Playback window has been closed, abort"
        n255 = event-data() -> ()  [unwired: 1 in, 4 out]
        n256 = local write "Rec Mode"(w402) -> ()
        n257 = global write "WPI_DashboardLogging Global.vi" "Recording"(w402) -> ()
      }
      event Panel Close {
        # "Abort playback window and ourself"
        n258 = event-data() -> ()  [unwired: 1 in, 4 out]
        n259 = invoke class="VI" method="FP.Close"(reference=w407) -> (reference out=w406:refnum<vi>)  [unwired: 2 in, 2 out]
        n260 = invoke class="VI" method="Abort VI"(reference=w406) -> (error out=w405:errorcluster)  [unwired: 2 in, 2 out]
        n261 = invoke class="VI" method="Abort VI"(error in=w405) -> ()  [unwired: 2 in, 3 out]
      }
      event "Vision": Value Change {
        # "Enable/Disable Compression slider.\nHW USB is hard-coded into the camera"
        n262 = event-data() -> ("NewVal"=w413:u16)  [unwired: 1 in]
        n263 = Equal?(x=w413, y=u32 2 ("milliseconds to wait")) -> (x = y?=w411:bool)
        n264 = Select(t=T23."Disabled and Grayed Out" ("Disabled"), s=w411, f=T23."Enabled" ("Disabled")) -> (s? t:f=w408:T23)
        n265 = property on="Compression" class="Slide (strict)"("DisabledEnum"=w408) -> ()  [unwired: 2 in, 2 out]
      }
    }
  }
  n266 = while {
    tunnel: w48 -> [w416]
    i -> [w419]
    stop <- FALSE stop-if-true
    n267 = Wait (ms)(milliseconds to wait=u32 100) -> ()  [unwired: 1 out]
    n268 = case shown="\"Playback\"" "Rec Mode" {
      tunnel: w419 -> [_ _ w434]
      tunnel: [u32 2829099 ("Base Color") u32 11141120 ("Target Color") w423] -> w415
      frame "Stop", Default {
        # "Reset the color, extra updates don't cost much"
      }
      frame "Record" {
      }
      frame "Playback" {
        # "Playback"
        n269 = Quotient & Remainder(x=w434, y=u32 50 ("milliseconds to wait")) -> (x-y*floor(x/y)=w430:u32)  [unwired: 1 out]
        n270 = Divide(x=w430, y=u32 50 ("milliseconds to wait")) -> (x/y=w427:dbl)
        n271 = Multiply(x=6.283185307179586, y=w427) -> (x*y=w432:dbl)
        n272 = Sine(x=w432) -> (sin(x)=w431:dbl)
        n273 = Absolute Value(x=w431) -> (abs(x)=w424:dbl)
        n274 = call "Interpolate RGB Color.vi"("Proportion"=w424, "Target Color"=u32 30976, "Base Color"=u32 2829099) -> ("Result Color"=w423:u32)  [unwired: 8 in]
      }
    }
    n275 = property class="Pane"(reference=w416, "PaneColor"=w415) -> ()  [unwired: 1 in, 2 out]
  }
  n276 = TCP Create Listener(10:u16 1741 ("timeout ms (25000)")) -> (3:w11:refnum<k5>)  [unwired: 4 in, 2 out]
  n277 = while {
    tunnel: w11 -> [w436]
    stop <- FALSE stop-if-true
    n278 = TCP Wait On Listener(11:w436) -> (4:w435:refnum<k5>)  [unwired: 3 in, 4 out]
    n279 = local write "TCP"(w435) -> ()
  }
  n280 = property on="On/Off" class="Bool (strict)"("Visible"=w16) -> ()  [unwired: 2 in, 2 out]
  n281 = property on="Motor" class="Clust (strict)"("Visible"=w16) -> ()  [unwired: 2 in, 2 out]
  n282 = property on="Progress" class="Clust (strict)"("Visible"=w16) -> ()  [unwired: 2 in, 2 out]
  n283 = property on="Test Ring" class="Ring (strict)"("Visible"=w16) -> ()  [unwired: 2 in, 2 out]
  n284 = property on="Rev/Fwd" class="Clust (strict)"("Visible"=w16) -> ()  [unwired: 2 in, 2 out]
  n285 = property on="Camera Settings" class="Clust (strict)"("Visible"=w16) -> ()  [unwired: 2 in, 2 out]
  n286 = local write "DB Camera Config"(w16) -> ()
  n287 = global write "WPI_DashboardLogging Global.vi" "Recording"(w42) -> ()
  n288 = local write "Rec Mode"(w42) -> ()
  n289 = call-poly <vilib>:"SD Write Value.vi"("String"="Auto Mode", "Name"="Autonomous Mode") -> ()  [unwired: 8 in, 2 out]
  n290 = Build Array("Shifting time (Initial)", "Desired Arm height (Lowered)", "Arm Speed", "Turning Speed", "Move Speed", "Shifting Speed", "Desired Arm height (Lift)") -> (w8:dbl[])
  n291 = call-poly <vilib>:"SD Write Value.vi"("Numeric Array"=w8) -> ()  [unwired: 9 in, 2 out]
